vi "IO_18v7Scaling.vi"(6 "!Enabled":bool, 8 "Pump Params":T1={"Empty Inches"=0.0, "Full Inches"=0.0, "RNG_SLOW"=0.5, "RNG_CREEP"=0.007, "RNG_STOP "=0.002, "VISA resource name"="COM4", "SPD_SLOW"=0, "SPD_CREEP"=0, "SPD_FAST"=0, "Zero template"=path "C:/AllenProjects/PWC-OLS/$Calibrtation/CAL_Level_RnR_241105.xlsx", "zero  Settle sec"=0.0} {"RNG_STOP" format="%#_13g"; "RNG_CREEP" format="%#_13g"; "RNG_SLOW" format="%#_13g"}, 9 "Drain":bool, 10 "Fill":bool, 11 "Pump Speed":T2) -> (1 "Speed Out":i32, 3 "Driver Signals":T3)   [LabVIEW 2024]
uses:
  Control Definitions/DEF_18v7DriverInputs.ctl
  Control Definitions/Def_PumpSpeed.ctl
  Control Definitions/DEF_PumpParams.ctl
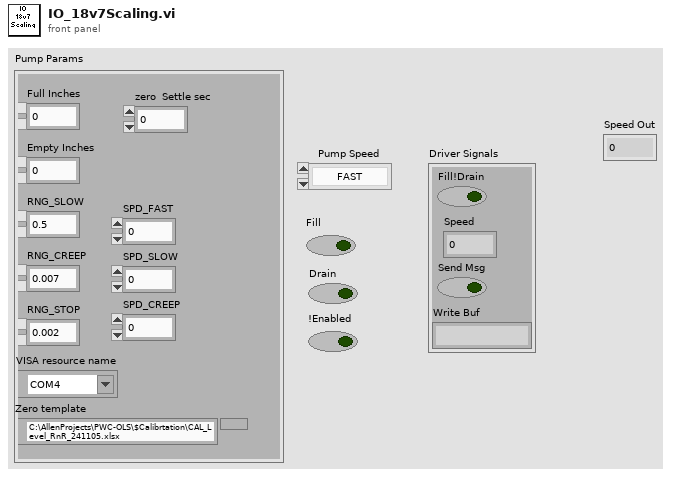
[diagram p1: front panel]
types:
  T1 = typedef "DEF_PumpParams.ctl" = cluster{"Empty Inches":dbl, "Full Inches":dbl, "RNG_SLOW":dbl, "RNG_CREEP":dbl, "RNG_STOP ":dbl, "VISA resource name":refnum<visa-resource-name>, "SPD_SLOW":i32, "SPD_CREEP":i32, "SPD_FAST":i32, "Zero template":path, "zero  Settle sec":dbl}
  T2 = typedef "Def_PumpSpeed.ctl" = enum16{"FAST", "SLOW", "CREEP", "STOP"}
  T3 = typedef "DEF_18v7DriverInputs.ctl" = cluster{"Fill!Drain":bool, "Speed":i16, "Send Msg":bool, "Write Buf":string}
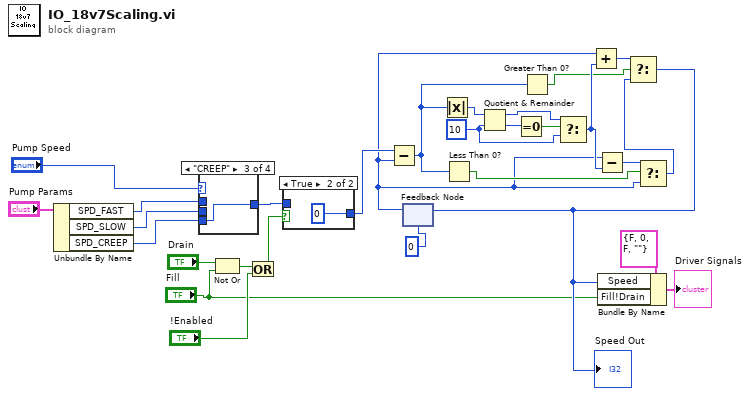
[diagram p0: block diagram]
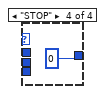
[diagram p5: hidden frame]
diagram:
  w21 = 10
  n1 = Unbundle By Name("Pump Params") -> ("SPD_FAST"=w8:i32, "SPD_SLOW"=w7:i32, "SPD_CREEP"=w6:i32)
  n2 = case shown="\"CREEP\"" "Pump Speed" {
    tunnel: [w30 w31 w32 0] -> w26
    tunnel: w8 -> [w30 _ _ _]
    tunnel: w7 -> [_ w31 _ _]
    tunnel: w6 -> [_ _ w32 _]
    frame "FAST", Default {
    }
    frame "SLOW" {
    }
    frame "CREEP" {
    }
    frame "STOP" {
    }
  }
  n3 = Not Or(1:"Fill", 2:"Drain") -> (0:w5:bool)
  n4 = Or(x=w5, y="!Enabled") -> (x .or. y?=w4:bool)
  n5 = case shown="True" w4 {
    tunnel: w26 -> [w34 _]
    tunnel: [w34 0] -> w20
    frame False {
    }
    frame True {
    }
  }
  n6 = feedback #1(0) -> (w16:i32)
  n7 = Subtract(x=w20, y=w16) -> (x-y=w10:i32)
  n8 = Absolute Value(x=w10) -> (abs(x)=w11:i32)
  n9 = Less Than 0?(x=w10) -> (x < 0?=w17:bool)
  n10 = Quotient & Remainder(x=w11, y=w21) -> (x-y*floor(x/y)=w22:i32, floor(x/y)=w24:i32)
  n11 = Equal To 0?(x=w24) -> (x = 0?=w23:bool)
  n12 = Greater Than 0?(x=w10) -> (x > 0?=w14:bool)
  n13 = Select(t=w22, s=w23, f=w21) -> (s? t:f=w19:i32)
  n14 = Add(x=w16, y=w19) -> (x+y=w15:i32)
  n15 = Subtract(x=w16, y=w19) -> (x-y=w18:i32)
  n16 = Select(t=w18, s=w17, f=w16) -> (s? t:f=w13:i32)
  n17 = Select(t=w15, s=w14, f=w13) -> (s? t:f=w12:i32)
  "Speed Out" <- w12
  n18 = feedback-in #1(w12) -> ()
  n19 = Bundle By Name(cluster=T3 {"Fill!Drain"=FALSE, "Speed"=0, "Send Msg"=FALSE, "Write Buf"=""} ("Inputs"), "Speed"=w12, "Fill!Drain"="Fill") -> (→"Driver Signals":T3)
